vi "creadorOrden.vi"(10 "Array":string[](array[string])) -> (2 "Array 2":T1(array[ring]))   [LabVIEW 2016]
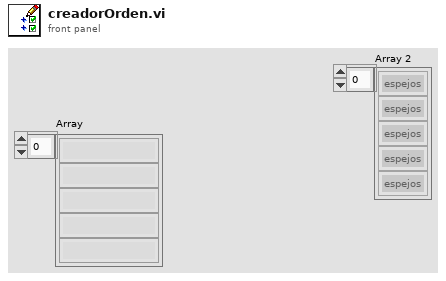
[diagram p1: front panel]
types:
  T1 = enum16{"espejos", "polarizador", "voltaje", "potenciometro ", "CCD", "lockin", "laser", "ninguno"}[]
  T2 = enum16{"espejos", "polarizador", "voltaje", "potenciometro ", "CCD", "lockin", "laser", "ninguno"}
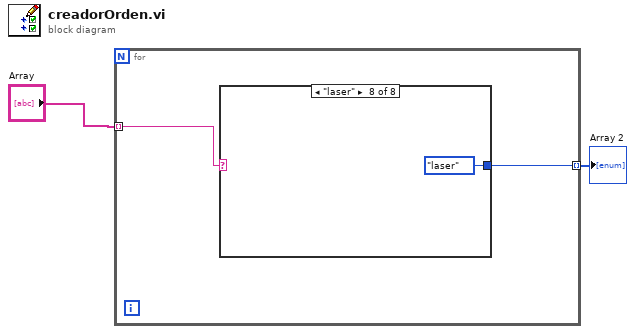
[diagram p0: block diagram]
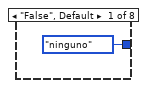
[diagram p2: hidden frame]
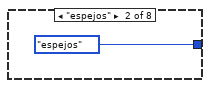
[diagram p3: hidden frame]
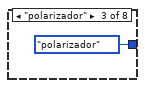
[diagram p4: hidden frame]
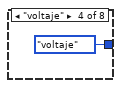
[diagram p5: hidden frame]
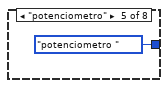
[diagram p6: hidden frame]
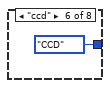
[diagram p7: hidden frame]
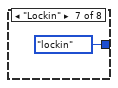
[diagram p8: hidden frame]
diagram:
  n1 = for {
    tunnel: "Array" -> [w4] mode=indexing
    tunnel: [w3] -> w1 mode=indexing
    n2 = case shown="\"laser\"" w4 {
      tunnel: [T2."ninguno" ("Enum") T2."espejos" ("Enum") T2."polarizador" ("Enum") T2."voltaje" ("Enum") T2."potenciometro " ("Enum") T2."CCD" ("Enum") T2."lockin" ("Enum") T2."laser" ("Enum")] -> w3
      frame "False", Default {
      }
      frame "espejos" {
      }
      frame "polarizador" {
      }
      frame "voltaje" {
      }
      frame "potenciometro" {
      }
      frame "ccd" {
      }
      frame "Lockin" {
      }
      frame "laser" {
      }
    }
  }
  "Array 2" <- w1
